vi "Convert J1939 ID to CAN Arb ID.vi"(0 "Priority":u8=6, 7 "PGN Fields":T1={"Reserved Bit"=0, "Data page"=0, "PDU Format"=254, "PDU Specific"=250}, 11 "Source Address":u8=27) -> (4 "ID":u32 format="%.0x", 8 "PGN":u32 format="%.0x")   [LabVIEW 2015, in "J1939 Addon Shared.lvlib" / "J1939 Utilities.lvlib"]
uses:
  J1939 Utilities.lvlib
  Types/PGN Fields Cluster.ctl
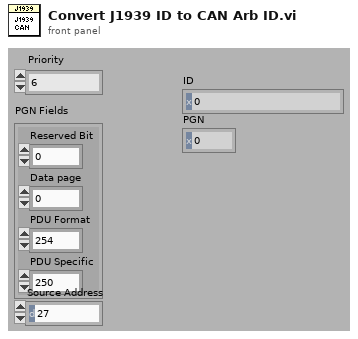
[diagram p1: front panel]
types:
  T1 = typedef "J1939 Addon Shared.lvlib/J1939 Utilities.lvlib/PGN Fields Cluster.ctl" = cluster{"Reserved Bit":u8, "Data page":u8, "PDU Format":u8, "PDU Specific":u8}
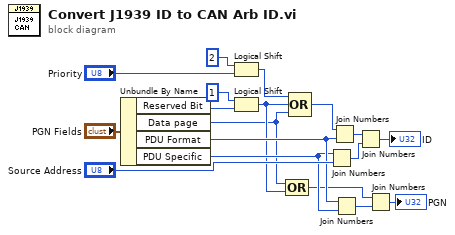
[diagram p0: block diagram]
diagram:
  n1 = Unbundle By Name("PGN Fields") -> ("Reserved Bit"=w16:u8, "Data page"=w2:u8, "PDU Format"=w7:u8, "PDU Specific"=w6:u8)
  n2 = Logical Shift(y=i8 2, x="Priority") -> (x << y=w8:u8)
  n3 = Logical Shift(y=i8 1, x=w16) -> (x << y=w3:u8)
  n4 = Compound Arithmetic op=OR(w2, w3) -> (w1:u8)
  n5 = Compound Arithmetic op=OR(w8, w3, w2) -> (w10:u8)
  n6 = Join Numbers(hi=w6, lo="Source Address") -> ((hi.lo)=w11:u16)
  n7 = Join Numbers(hi=w10, lo=w7) -> ((hi.lo)=w9:u16)
  n8 = Join Numbers(hi=w7, lo=w6) -> ((hi.lo)=w5:u16)
  n9 = Join Numbers(hi=w9, lo=w11) -> ((hi.lo)=→"ID":u32)
  n10 = Join Numbers(hi=w1, lo=w5) -> ((hi.lo)=→"PGN":u32)
